vi "CHECK NEO INVERT.vi"(0 "SparkMAX MotorControlDeviceRef in":T1, 1 "Invert mode?":bool, 3 "input1":dbl, 4 "input2":dbl) -> (14 "SparkMAX MotorControlDeviceRef out":T1, 15 "matched?":bool, 16 "multiplier":dbl, 17 "output 1":dbl, 18 "output 2":dbl)   [LabVIEW 2020]
uses:
  <vilib>/Rock Robotics/WPI/MotorControl/WPI_MotorControlDeviceRef.ctl
  <vilib>/Rock Robotics/WPI/MotorControl/WPI_MotorControlType.ctl
  <vilib>/Rock Robotics/SystemInterfaces/DIO/FPGA_DIOPWMChannel.ctl
  <vilib>/Rock Robotics/WPI/PWM/WPI_PWMDeadband.ctl
  <vilib>/Rock Robotics/SystemInterfaces/DIO/FPGA_DIOChannel.ctl
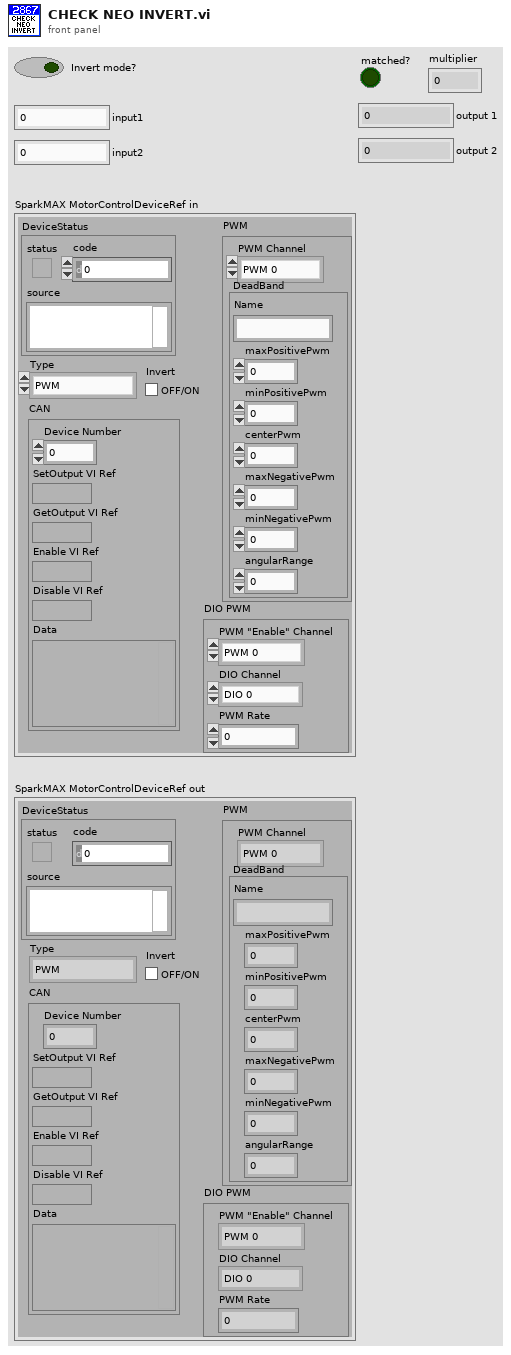
[diagram p1: front panel]
types:
  T1 = typedef "WPI_MotorControlDeviceRef.ctl" = cluster{"DeviceStatus":errorcluster, "Type":T2, "PWM":cluster{"PWM Channel":T3, "DeadBand":T4}, "CAN":cluster{"Device Number":u8, "SetOutput VI Ref":variant, "GetOutput VI Ref":variant, "Enable VI Ref":variant, "Disable VI Ref":variant, "Data":variant}, "Invert":bool, "DIO PWM":cluster{"PWM \"Enable\" Channel":T3, "DIOChannel":T5, "PWM Rate":dbl}}
  T2 = typedef "WPI_MotorControlType.ctl" = enum16{"PWM", "CAN", "DIO PWM"}
  T3 = typedef "FPGA_DIOPWMChannel.ctl" = enum8{"PWM 0", "PWM 1", "PWM 2", "PWM 3", "PWM 4", "PWM 5", "PWM 6", "PWM 7", "PWM 8", "PWM 9", "PWM MXP 0", "PWM MXP 1", "PWM MXP 2", "PWM MXP 3", "PWM MXP 4", "PWM MXP 5", "PWM MXP 6", "PWM MXP 7", "PWM MXP 8", "PWM MXP 9", "Invalid"}
  T4 = typedef "WPI_PWMDeadband.ctl" = cluster{"Name":string, "maxPositivePwm":i32, "minPositivePwm":i32, "centerPwm":i32, "maxNegativePwm":i32, "minNegativePwm":i32, "angularRange":u16}
  T5 = typedef "FPGA_DIOChannel.ctl" = enum8{"DIO 0", "DIO 1", "DIO 2", "DIO 3", "DIO 4", "DIO 5", "DIO 6", "DIO 7", "DIO 8", "DIO 9", "DIO MXP 0", "DIO MXP 1", "DIO MXP 2", "DIO MXP 3", "DIO MXP 4", "DIO MXP 5", "DIO MXP 6", "DIO MXP 7", "DIO MXP 8", "DIO MXP 9", "DIO MXP 10", "DIO MXP 11", "DIO MXP 12", "DIO MXP 13", "DIO MXP 14", "DIO MXP 15", "SPI Port CS1", "SPI Port CS2", "SPI Port CS3", "SPI Port MISO", "SPI Port MOSI", "Invalid"}
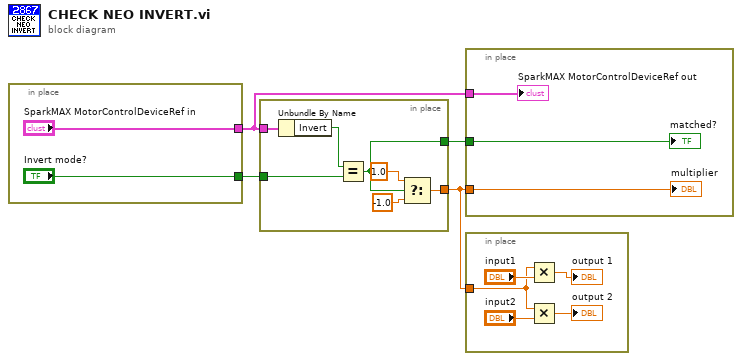
[diagram p0: block diagram]
diagram:
  n1 = in-place {
    in-place-border: ["Invert mode?"] -> w3
    in-place-border: ["SparkMAX MotorControlDeviceRef in"] -> w1
  }
  n2 = in-place {
    in-place-border: [w11] -> w4
    in-place-border: w3 -> [w10]
    in-place-border: w1 -> [w8]
    in-place-border: [w7] -> w2
    n3 = Unbundle By Name(w8) -> ("Invert"=w9:bool)
    n4 = Equal?(x=w9, y=w10) -> (x = y?=w11:bool)
    n5 = Select(t=1.0, s=w11, f=-1.0) -> (s? t:f=w7:dbl)
  }
  n6 = in-place {
    in-place-border: w4 -> [w16]
    in-place-border: w2 -> [w15]
    in-place-border: w1 -> [w14]
    "matched?" <- w16
    "multiplier" <- w15
    "SparkMAX MotorControlDeviceRef out" <- w14
  }
  n7 = in-place {
    in-place-border: w2 -> [w20]
    n8 = Multiply(x=w20, y="input1") -> (x*y=→"output 1":dbl)
    n9 = Multiply(x=w20, y="input2") -> (x*y=→"output 2":dbl)
  }
